vi "Intake Process.vi"   [LabVIEW 2013]
uses:
  Intake Global.vi
types:
  T1 = typedef "WPI_RelayValue.ctl" = enum16{"Off", "On", "Forward", "Reverse"}
  T2 = typedef "WPI_SolenoidValue.ctl" = enum16{"Off", "On", "Forward", "Reverse"}
  T3 = cluster{"Arm State":bool, "Gripper Out":bool, "Gripper Execution":T1, "Arm Execution":T2, "Gripper In":bool}
  T4 = cluster{"Arm State":bool, "Gripper In":bool, "Gripper Execution":T1, "Arm Execution":T2, "Gripper Out":bool}
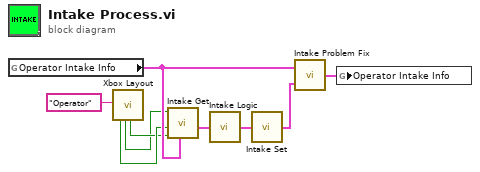
[diagram p0: block diagram]
diagram:
  n1 = global read "Intake Global.vi" "Operator Intake Info"() -> (w5:T3)
  n2 = call "Xbox Layout.vi"("Joystick Name"="Operator") -> ("A"=w3:bool, "B"=w1:bool, "X"=w2:bool)  [unwired: 3 in, 13 out]
  n3 = call "Intake Get.vi"("Operator Intake In"=w5, "Gripper"=w2, "Gripper In"=w3, "Arm State"=w1) -> ("Operator Intake Out"=w7:T3)  [unwired: 6 in, 1 out]
  n4 = call "Intake Logic.vi"("Operator Intake In"=w7) -> ("Operator Intake Out"=w8:T3)
  n5 = call "Intake Set.vi"("Operator Intake In"=w8) -> ("Operator Intake Out"=w9:T4)
  n6 = call "Intake Problem Fix.vi"("Operator Intake Modified"=w9, "Operator Intake Original"=w5) -> ("Operator Intake Fixed"=w6:T3)
  n7 = global write "Intake Global.vi" "Operator Intake Info"(w6) -> ()
